vi "example_llm_ollama_unit_test_1.vi"() -> ()   [LabVIEW 2020]
uses:
  llm_ollama_chatmodels/llm_ollama_chatmodels.lvclass
  message_text/message_text.lvclass
  D:/lv_llm/labview-llm-libraries/src/models/abstract_message_base/abstract_message_base.lvclass
  message_text/message.ctl
panel:
  in  "Ollama URL":string="http://localhost:11434"
  in  "Messages":cluster{"role":string, "text":string}[](array[cluster])=[{"role"="system", "text"="Act as a math teacher and guide the student in solving the problem. You should not solve the problem. Always answer in single line."}, {"role"="user", "text"="What is x in the equation 2x + 3 = 5  ?"}]
  out "error out":errorcluster
  in  "model_name":string(combo)="tinyllama"
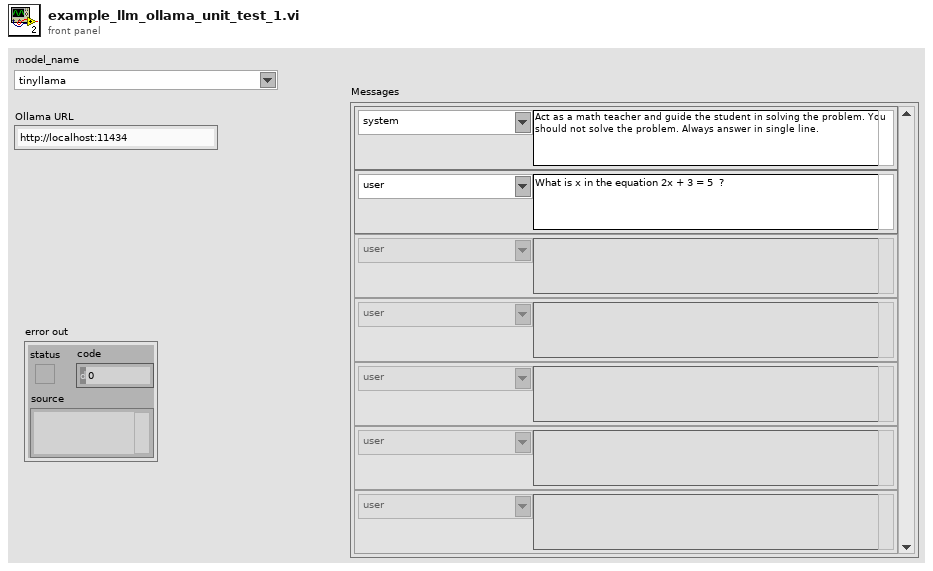
[diagram p1: front panel]
types:
  T1 = typedef "message_text.lvclass/message.ctl" = cluster{"role":string, "content":string[]}
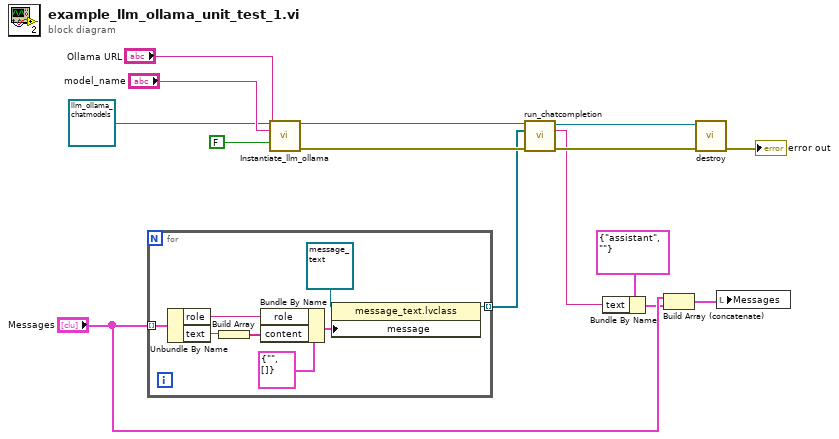
[diagram p0: block diagram]
diagram:
  n1 = for {
    tunnel: "Messages" -> [w21] mode=indexing
    tunnel: [w22] -> w9 mode=indexing
    n2 = Unbundle By Name(w21) -> ("role"=w19:string, "text"=w17:string)
    n3 = Build Array(w17) -> (w16:string[])
    n4 = Bundle By Name(cluster=T1 {"role"="", "content"=[]} ("message"), "role"=w19, "content"=w16) -> (w18:T1)
    n5 = property class="message_text.lvclass"(reference=refnum<class "message_text.lvclass"> refnum ("message_text.lvclass"), "message"=w18) -> (reference out=w22:refnum<class "message_text.lvclass">)  [unwired: 1 in, 1 out]
  }
  n6 = call "Instantiate_llm_ollama.vi"("llm_openai in"=refnum<class "llm_ollama_chatmodels.lvclass"> refnum ("llm_ollama_chatmodels.lvclass"), "model_name"="model_name", "Ollama URL"="Ollama URL", "EnableStreaming"=FALSE) -> ("llm_openai out"=w15:refnum<class "llm_ollama_chatmodels.lvclass">, "error out"=w14:errorcluster)  [unwired: 10 in]
  n7 = call-dynamic "run_chatcompletion.vi"("chatcompletion_llm_interface in"=w15, "Messages"=w9, "error in (no error)"=w14) -> ("chatcompletion_llm_interface out"=w12:refnum<class "llm_ollama_chatmodels.lvclass">, "chat response"=w5:string, "error out"=w11:errorcluster)  [unwired: 10 in]
  n8 = Bundle By Name(cluster=cluster{"role":string, "text":string} {"role"="assistant", "text"=""} ("message"), "text"=w5) -> (w4:cluster{"role":string, "text":string})
  n9 = Build Array (concatenate)("Messages", w4) -> (w7:cluster{"role":string, "text":string}[])
  n10 = call-dynamic "destroy.vi"("error in (no error)"=w11, "abstract_llm_base in"=w12) -> ("error out"=→"error out":errorcluster)  [unwired: 8 in, 1 out]
  n11 = local write "Messages"(w7) -> ()
